vi "classes.vi"(0 "HB_Factory":refnum<class "HB_Factory.lvclass">, 1 "className":string, 5 "error in (no error)":errorcluster) -> (14 "dup HB_Factory":refnum<class "HB_Factory.lvclass">, 16 "Object":refnum<class>, 19 "error out":errorcluster)   [LabVIEW 2009, in "HB_BaseClass_Examples.lvlib" / "HB_Factory.lvclass"]
doc: "This dynamaic dispatch VI contains constant objects of all classes that can be produced by HB_Factory.\n\nChild classes can override it to define additional classes."
uses:
  HB_Factory.lvclass
  HB_Simple/HB_Simple.lvclass
  HB_Simple/Visitors/Add/HB_Simple_Add.lvclass
  HB_Simple/Visitors/Decrement/HB_Simple_Decrement.lvclass
  HB_Simple/Visitors/Increment/HB_Simple_Increment.lvclass
  HB_Composite/HB_Society/HB_Society.lvclass
  lib.lib/HGF_LVC/HGF_BaseClasses/HGF_Factory/HGF_Factory.lvclass
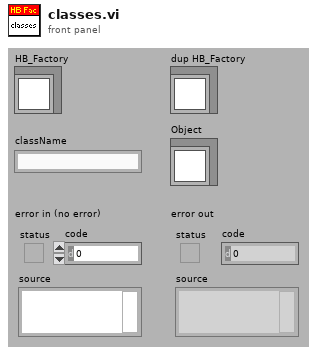
[diagram p1: front panel]
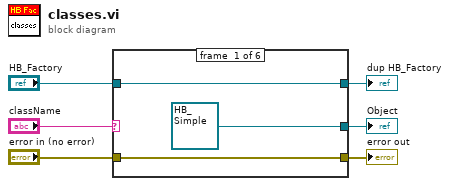
[diagram p0: block diagram]
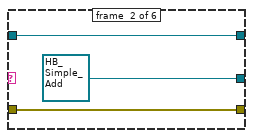
[diagram p2: hidden frame]
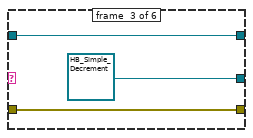
[diagram p3: hidden frame]
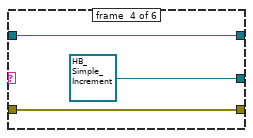
[diagram p4: hidden frame]
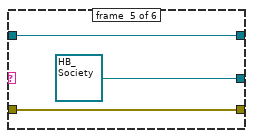
[diagram p5: hidden frame]
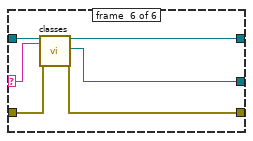
[diagram p6: hidden frame]
diagram:
  n1 = case shown="Default" "className" {
    selector: "className" -> [_ _ _ _ _ w22]
    tunnel: "HB_Factory" -> [w9 w12 w13 w18 w21 w27]
    tunnel: "error in (no error)" -> [w8 w11 w14 w17 w20 w26]
    tunnel: [w9 w12 w13 w18 w21 w25] -> w4
    tunnel: [refnum<class "HB_Simple.lvclass"> refnum ("HB_Simple.lvclass") refnum<class "HB_Simple_Add.lvclass"> refnum ("HB_HGF_Test.lvlib:HB_Simple_Add.lvclass") refnum<class "HB_Simple_Decrement.lvclass"> refnum ("HB_Simple_Decrement.lvclass") refnum<class "HB_Simple_Increment.lvclass"> refnum ("HB_Simple_Increment.lvclass") refnum<class "HB_Society.lvclass"> refnum ("MySociety.lvclass") w24] -> w3
    tunnel: [w8 w11 w14 w17 w20 w23] -> w2
    frame #0 {
    }
    frame #1 {
    }
    frame #2 {
    }
    frame #3 {
    }
    frame #4 {
    }
    frame #5 {
      n2 = call-parent "classes.vi"("HGF_Factory"=w27, "className"=w22, "error in (no error)"=w26) -> ("HGF_Factory dup"=w25:refnum<class "HB_Factory.lvclass">, "Object"=w24:refnum<class>, "error out"=w23:errorcluster)  [unwired: 14 out]
    }
  }
  "error out" <- w2
  "dup HB_Factory" <- w4
  "Object" <- w3
